vi "FTW-TransferClient-Cancel.vi"(0 "Transfer Client":refnum<class "FTW-TransferClient.lvclass">, 11 "error in":errorcluster) -> (4 "Transfer Client out":refnum<class "FTW-TransferClient.lvclass">, 15 "error out":errorcluster)   [LabVIEW 2012, in "FTW-TransferClient.lvclass"]
uses:
  FTW-TransferClient.lvclass
panel:
  # "Inputs"
  # "Outputs"
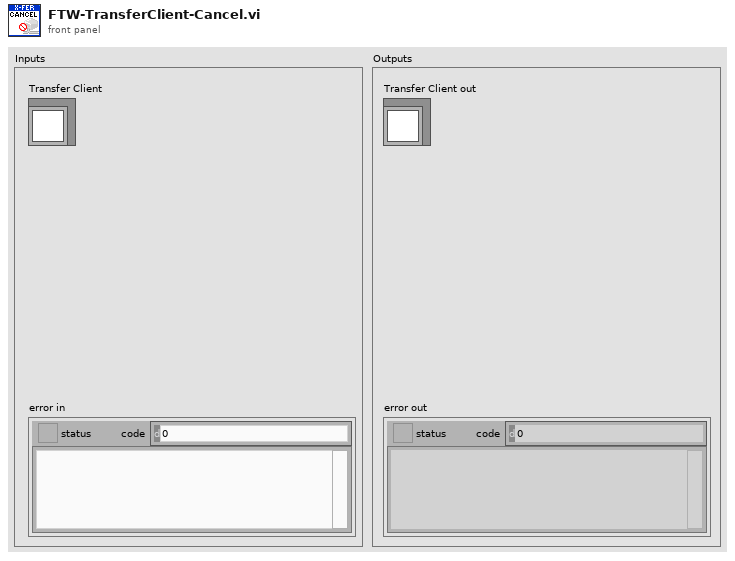
[diagram p1: front panel]
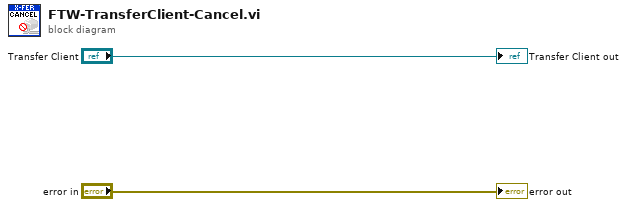
[diagram p0: block diagram]
diagram:
  "error out" <- "error in"
  "Transfer Client out" <- "Transfer Client"
